vi "Pulse_Width-NI.AI.vi"(6 "TestMode":enum16{"测试脉冲宽度或上升边沿", "测试下降边沿"}(ring), 7 "input terminal configuration":i32(ring)=-1 caption="输入接线端配置" items=["默认"=-1, "RSE"=10083, "NRSE"=10078, "差分"=10106, "伪差分"=12529], 8 "error in":errorcluster caption="错误输入", 9 "Trigger_Voltage(VDC)":dbl, 10 "AI Channel":T1(ring), 11 "DAQmx设备名":tag) -> (0 "error out":errorcluster caption="错误输出", 1 "OSC.Trip":dbl[](array[numeric]), 2 "Times":u32, 3 "ok?":bool)   [LabVIEW 2012, in "Lib_UEL.ATE.lvlib" / "Lib_PCI6221.lvlib"]
uses:
  Lib_PCI6221.lvlib
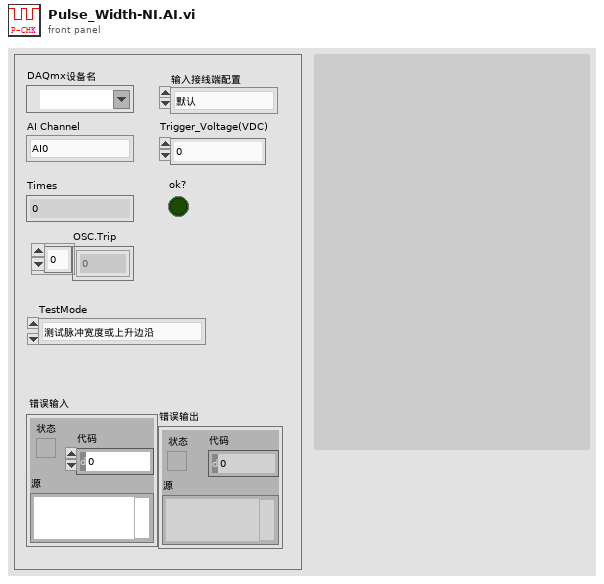
[diagram p1: front panel]
types:
  T1 = enum16{"AI0", "AI1", "AI2", "AI3", "AI4", "AI5", "AI6", "AI7", "AI8", "AI9", "AI10", "AI11", "AI12", "AI13", "AI14", "AI15"}
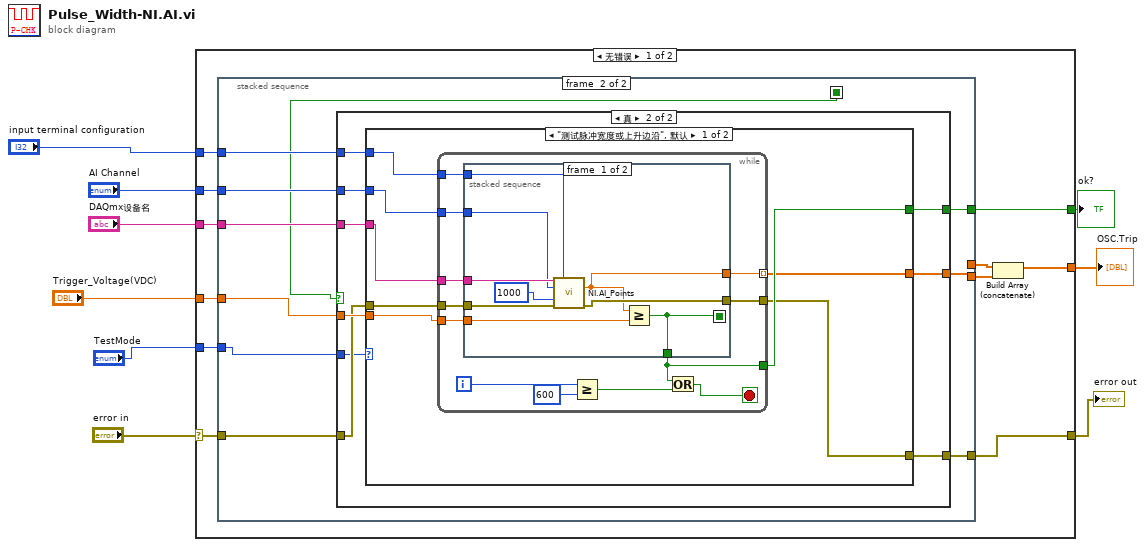
[diagram p0: block diagram]
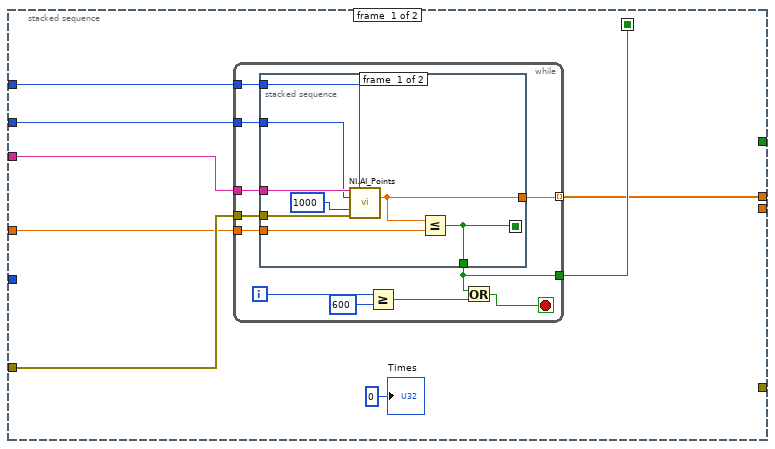
[diagram p2: hidden frame]
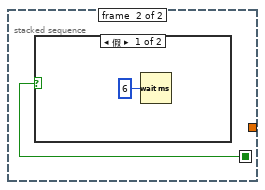
[diagram p3: hidden frame]
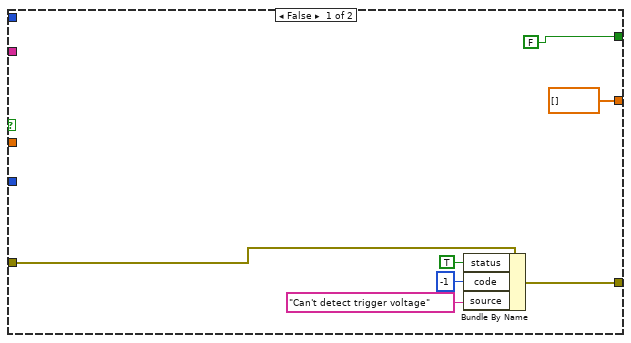
[diagram p5: hidden frame]
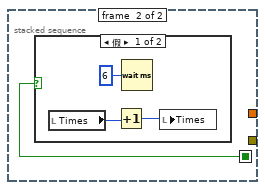
[diagram p6: hidden frame]
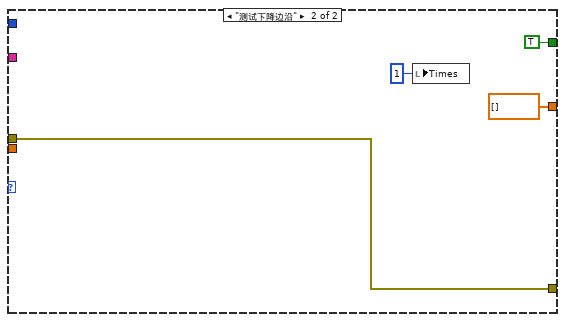
[diagram p8: hidden frame]
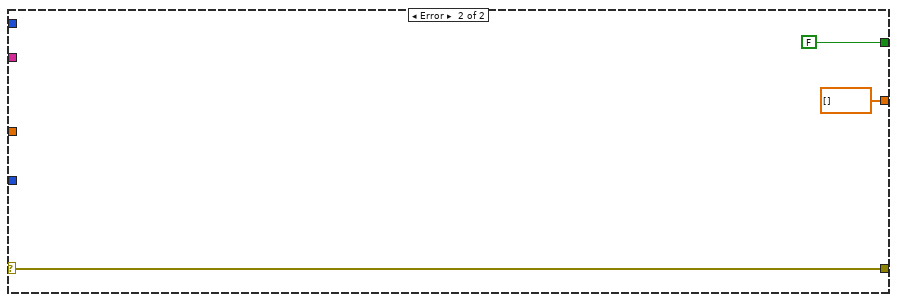
[diagram p9: hidden frame]
diagram:
  n1 = case shown="无错误" "error in" {
    selector: "error in" -> [w19 w115]
    tunnel: "DAQmx设备名" -> [w20 _]
    tunnel: [w15 w115] -> w8
    tunnel: "input terminal configuration" -> [w18 _]
    tunnel: "AI Channel" -> [w17 _]
    tunnel: "Trigger_Voltage(VDC)" -> [w16 _]
    tunnel: [w14 FALSE ("ok?")] -> w4
    tunnel: [w11 dbl[] []] -> w2
    tunnel: "TestMode" -> [w10 _]
    frame No Error {
      n2 = stacked-sequence {
        seq-local: [w23 _] -> [_ w51]
        tunnel: w20 -> [w28 w54]
        tunnel: w19 -> [w27 w59]
        tunnel: w18 -> [w26 w57]
        tunnel: w17 -> [w25 w56]
        tunnel: w16 -> [w24 w55]
        tunnel: [_ w58] -> w15
        tunnel: [_ w53] -> w14
        tunnel: [w21 _] -> w13
        tunnel: [_ w52] -> w12
        tunnel: w10 -> [_ w50]
        frame #0 {
          n3 = while {
            tunnel: w28 -> [w39]
            tunnel: w27 -> [w38]
            tunnel: w26 -> [w37]
            tunnel: w25 -> [w36]
            tunnel: w24 -> [w35]
            tunnel: [w30] -> w23
            tunnel: [w29] -> w21 mode=indexing
            i -> [w34]
            stop <- w31 stop-if-true
            n4 = stacked-sequence {
              seq-local: [w42 _] -> [_ w48]
              tunnel: w39 -> [w47 _]
              tunnel: w38 -> [w46 _]
              tunnel: w37 -> [w45 _]
              tunnel: w36 -> [w44 _]
              tunnel: w35 -> [w43 _]
              tunnel: [w42 _] -> w30
              tunnel: [w40 _] -> w29
              frame #0 {
                n5 = call "NI.AI_Points.vi"("DAQmx设备名"=w47, "input terminal configuration"=w45, "AI Channel"=w44, "SignalRate"=u32 1000, "error in"=w46) -> ("RMS(VDC)"=w40:dbl)  [unwired: 4 in, 6 out]
                n6 = Less Or Equal?(x=w40, y=w43) -> (x <= y?=w42:bool)
              }
              frame #1 {
                n7 = case shown="假" w48 {
                  frame False {
                    n8 = Wait (ms)(milliseconds to wait=u32 6 ("等待时间（毫秒）")) -> ()  [unwired: 1 out]
                  }
                  frame True {
                  }
                }
              }
            }
            n9 = Greater Or Equal?(x=w34, y=600) -> (x >= y?=w32:bool)
            n10 = Or(x=w30, y=w32) -> (x .or. y?=w31:bool)
          }
          "Times" <- u32 0 ("Times")
        }
        frame #1 {
          n11 = case shown="真" w51 {
            tunnel: w59 -> [w66 w72]
            tunnel: [w65 w69] -> w58
            tunnel: w57 -> [_ w75]
            tunnel: w56 -> [_ w74]
            tunnel: w55 -> [_ w73]
            tunnel: w54 -> [_ w71]
            tunnel: [FALSE ("ok?") w70] -> w53
            tunnel: [dbl[] [] w68] -> w52
            tunnel: w50 -> [_ w67]
            frame False {
              n12 = Bundle By Name(cluster=w66, "status"=TRUE, "code"=-1, "source"="Can't detect trigger voltage") -> (w65:errorcluster)
            }
            frame True {
              n13 = case shown="\"测试脉冲宽度或上升边沿\", 默认" w67 {
                tunnel: w75 -> [w83 _]
                tunnel: w74 -> [w82 _]
                tunnel: w73 -> [w81 _]
                tunnel: w72 -> [w80 w110]
                tunnel: w71 -> [w79 _]
                tunnel: [w78 TRUE] -> w70
                tunnel: [w77 w110] -> w69
                tunnel: [w76 dbl[] []] -> w68
                frame "测试脉冲宽度或上升边沿", Default {
                  n14 = while {
                    tunnel: w79 -> [w95]
                    tunnel: w80 -> [w94]
                    tunnel: w83 -> [w93]
                    tunnel: w82 -> [w92]
                    tunnel: w81 -> [w91]
                    tunnel: [w86] -> w78
                    tunnel: [w85] -> w77
                    tunnel: [w84] -> w76 mode=indexing
                    i -> [w90]
                    stop <- w87 stop-if-true
                    n15 = stacked-sequence {
                      seq-local: [w99 _] -> [_ w105]
                      tunnel: w95 -> [w104 _]
                      tunnel: w94 -> [w103 _]
                      tunnel: w93 -> [w102 _]
                      tunnel: w92 -> [w101 _]
                      tunnel: w91 -> [w100 _]
                      tunnel: [w99 _] -> w86
                      tunnel: [w97 _] -> w85
                      tunnel: [w96 _] -> w84
                      frame #0 {
                        n16 = call "NI.AI_Points.vi"("DAQmx设备名"=w104, "input terminal configuration"=w102, "AI Channel"=w101, "SignalRate"=u32 1000, "error in"=w103) -> ("RMS(VDC)"=w96:dbl, "error out"=w97:errorcluster)  [unwired: 4 in, 5 out]
                        n17 = Greater Or Equal?(x=w96, y=w100) -> (x >= y?=w99:bool)
                      }
                      frame #1 {
                        n18 = case shown="假" w105 {
                          frame False {
                            n19 = local read "Times"() -> (w107:u32)
                            n20 = Increment(x=w107) -> (x+1=w106:u32)
                            n21 = Wait (ms)(milliseconds to wait=u32 6 ("等待时间（毫秒）")) -> ()  [unwired: 1 out]
                            n22 = local write "Times"(w106) -> ()
                          }
                          frame True {
                          }
                        }
                      }
                    }
                    n23 = Greater Or Equal?(x=w90, y=600) -> (x >= y?=w88:bool)
                    n24 = Or(x=w86, y=w88) -> (x .or. y?=w87:bool)
                  }
                }
                frame "测试下降边沿" {
                  n25 = local write "Times"(u32 1 ("Times")) -> ()
                }
              }
            }
          }
        }
      }
      n26 = Build Array (concatenate)(w13, w12) -> (w11:dbl[])
    }
    frame Error {
    }
  }
  "error out" <- w8
  "ok?" <- w4
  "OSC.Trip" <- w2
